vi "Init Transport.vi"() -> (2 "Transport":refnum<class "Transport.lvclass">)   [LabVIEW 2025, in "jettl.lvlib" / "Transport.lvlib" / "Notifier.lvlib"]
uses:
  Notifier.lvlib
  Transport/Transport.lvclass
  Notifier Transport/Notifier Transport.lvclass
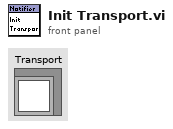
[diagram p1: front panel]
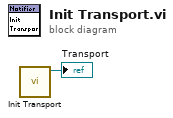
[diagram p0: block diagram]
diagram:
  n1 = call "Init Transport.vi"() -> ("Notifier Transport out"=→"Transport":refnum<class "Notifier Transport.lvclass">)  [unwired: 11 in]
